vi "Z900_navX_Internal_TimeoutCheck.vi"(2 "Allowed Error Count":i32=32, 3 "Valid Packet Reception Timeout (s)":dbl=2.0 format="%#_13g", 4 "Timout Status (in)":T1) -> (0 "TIMEOUT!":bool, 1 "Timout Status (out)":T1)   [LabVIEW 2015, in "navX Library v2.lvlib"]
uses:
  navX Library v2.lvlib
  TypeDefs/Z900_navX_InternalTimoutStatusTypeDef.ctl
  <vilib>/Rock Robotics/SystemInterfaces/Utilities/FPGA_UtilitiesRead LocalTime.vi
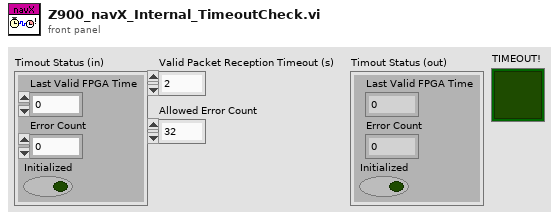
[diagram p1: front panel]
types:
  T1 = typedef "navX Library v2.lvlib/Z900_navX_InternalTimoutStatusTypeDef.ctl" = cluster{"Last Valid FPGA Time":dbl, "Error Count":i32, "Initialized":bool}
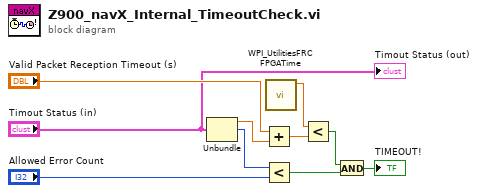
[diagram p0: block diagram]
diagram:
  n1 = Unbundle("Timout Status (in)") -> ("Last Valid FPGA Time"=w10:dbl, "Error Count"=w6:i32)  [unwired: 1 out]
  n2 = Add(x="Valid Packet Reception Timeout (s)", y=w10) -> (x+y=w8:dbl)
  n3 = Less?(x=w6, y="Allowed Error Count") -> (x < y?=w3:bool)
  n4 = call <vilib>:"WPI_UtilitiesFRC FPGATime.vi"() -> ("FPGA Time"=w7:dbl)  [unwired: 10 in, 1 out]
  n5 = Less?(x=w7, y=w8) -> (x < y?=w4:bool)
  n6 = And(x=w4, y=w3) -> (x .and. y?=→"TIMEOUT!":bool)
  "Timout Status (out)" <- "Timout Status (in)"
